vi "Periodic Tasks.vi"(8 "error in":errorcluster) -> ()   [LabVIEW 2017]
doc: "This VI runs in parallel to other robot code. It can contain as many user-defined periodic loops as you need. These can carry out PID or other sorts of timed response."
uses:
  <vilib>/Rock Robotics/WPI/Joystick/WPI_JoystickDeviceEnum.ctl
  <vilib>/Rock Robotics/WPI/Ultrasonic/WPI_SonarMB1010AnalogDeviceRef.ctl
  <vilib>/Rock Robotics/WPI/AnalogChannel/WPI_AnalogChannelDevRef.ctl
  <vilib>/Rock Robotics/SystemInterfaces/AI/FPGA_AIChannel.ctl
  <vilib>/Rock Robotics/WPI/ThirdParty/Sensors/ADIS16448 IMU/ADI_IMU_ADIS16448_IMUDevRef.ctl
  <vilib>/Rock Robotics/SystemInterfaces/spilib/spi_bus.ctl
  <vilib>/Rock Robotics/WPI/Utilities/WPI_GetSetVariantRefNum.vi
  <vilib>/Rock Robotics/WPI/Ultrasonic/WPI_SonarMB1010AnalogRefNum Registry Get.vi
  Robot Global Data.vi
  <vilib>/Rock Robotics/WPI/Ultrasonic/WPI_SonarMB1010AnalogGetRange.vi
  <vilib>/Rock Robotics/WPI/ThirdParty/Sensors/ADIS16448 IMU/ADIS16448_IMU.lvlib
panel:
  out "Current Faults":bool[](array[boolean])
  out "Battery Voltage Fault":bool
  out "Temperature Fault":bool
  out "Hardware Fault":bool
  out "IMU Angles Out":T1
  out "Z Angle":dbl
  out "Sonar Distance":dbl
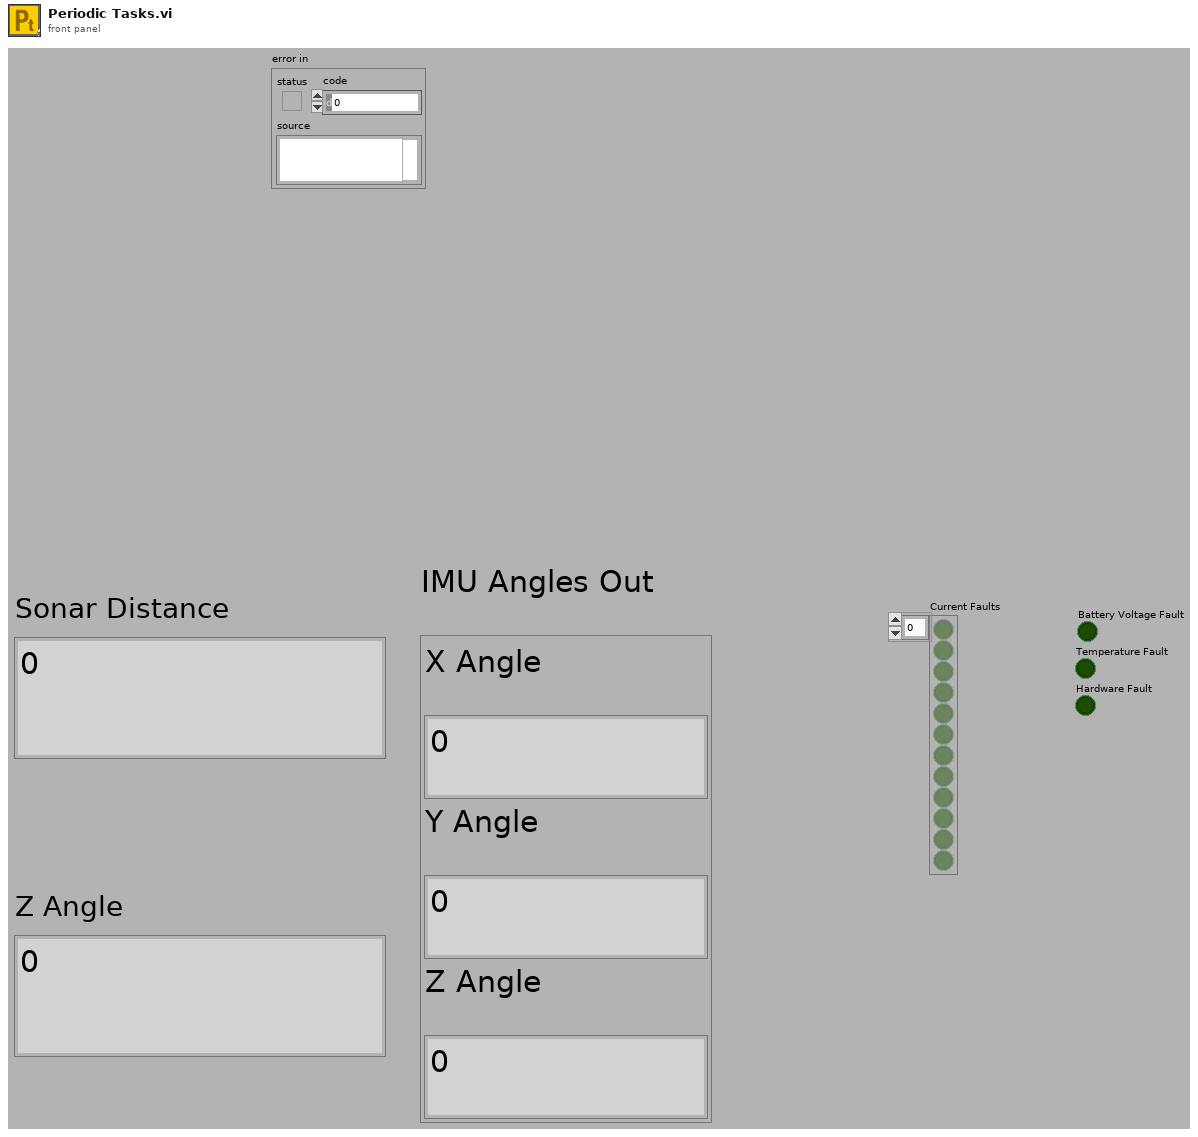
[diagram p1: front panel]
types:
  T1 = cluster{"X Angle":dbl, "Y Angle":dbl, "Z Angle":dbl}
  T2 = typedef "WPI_JoystickDeviceEnum.ctl" = enum16{"USB 0", "USB 1", "USB 2", "USB 3", "USB 4", "USB 5"}
  T3 = typedef "WPI_SonarMB1010AnalogDeviceRef.ctl" = cluster{"AIDeviceRef":T4, "Scaling factor (V/in)":dbl, "Average Bits":u8}
  T4 = typedef "WPI_AnalogChannelDevRef.ctl" = cluster{"DevStatus":errorcluster, "Analog Channel":T5}
  T5 = typedef "FPGA_AIChannel.ctl" = enum8{"AI 0", "AI 1", "AI 2", "AI 3", "AI MXP 0", "AI MXP 1", "AI MXP 2", "AI MXP 3", "Invalid"}
  T6 = typedef "ADIS16448_IMU.lvlib/ADI_IMU_ADIS16448_IMUDevRef.ctl" = cluster{"DevStatus":errorcluster, "Handle":i32, "SPI Bus":T7, "Device Found":bool, "Device Ready":bool, "Yaw Axis":enum16{"X", "Y", "Z"}, "AHRS Algorithm":enum16{"Complementary", "Madgwick"}, "Serial":u16, "Lot ID 2":u16, "Lot ID 1":u16, "Bytes Per Sample":u16, "Calibrate On Open?":bool}
  T7 = typedef "spi_bus.ctl" = enum16{"SPI On-Board, CS0", "SPI On-Board, CS1", "SPI On-Board, CS2", "SPI On-Board, CS3", "SPI MXP", "Invalid"}
  T8 = cluster{"Joystick 0":cluster{"Joystick 0":T2}, "Joystick 1":cluster{"Joystick 1":T2}, "Sonar":T3, "ADI IMU":T6}
  T9 = typedef "WPI_JoystickDevRef.ctl" = cluster{"Device":T2}
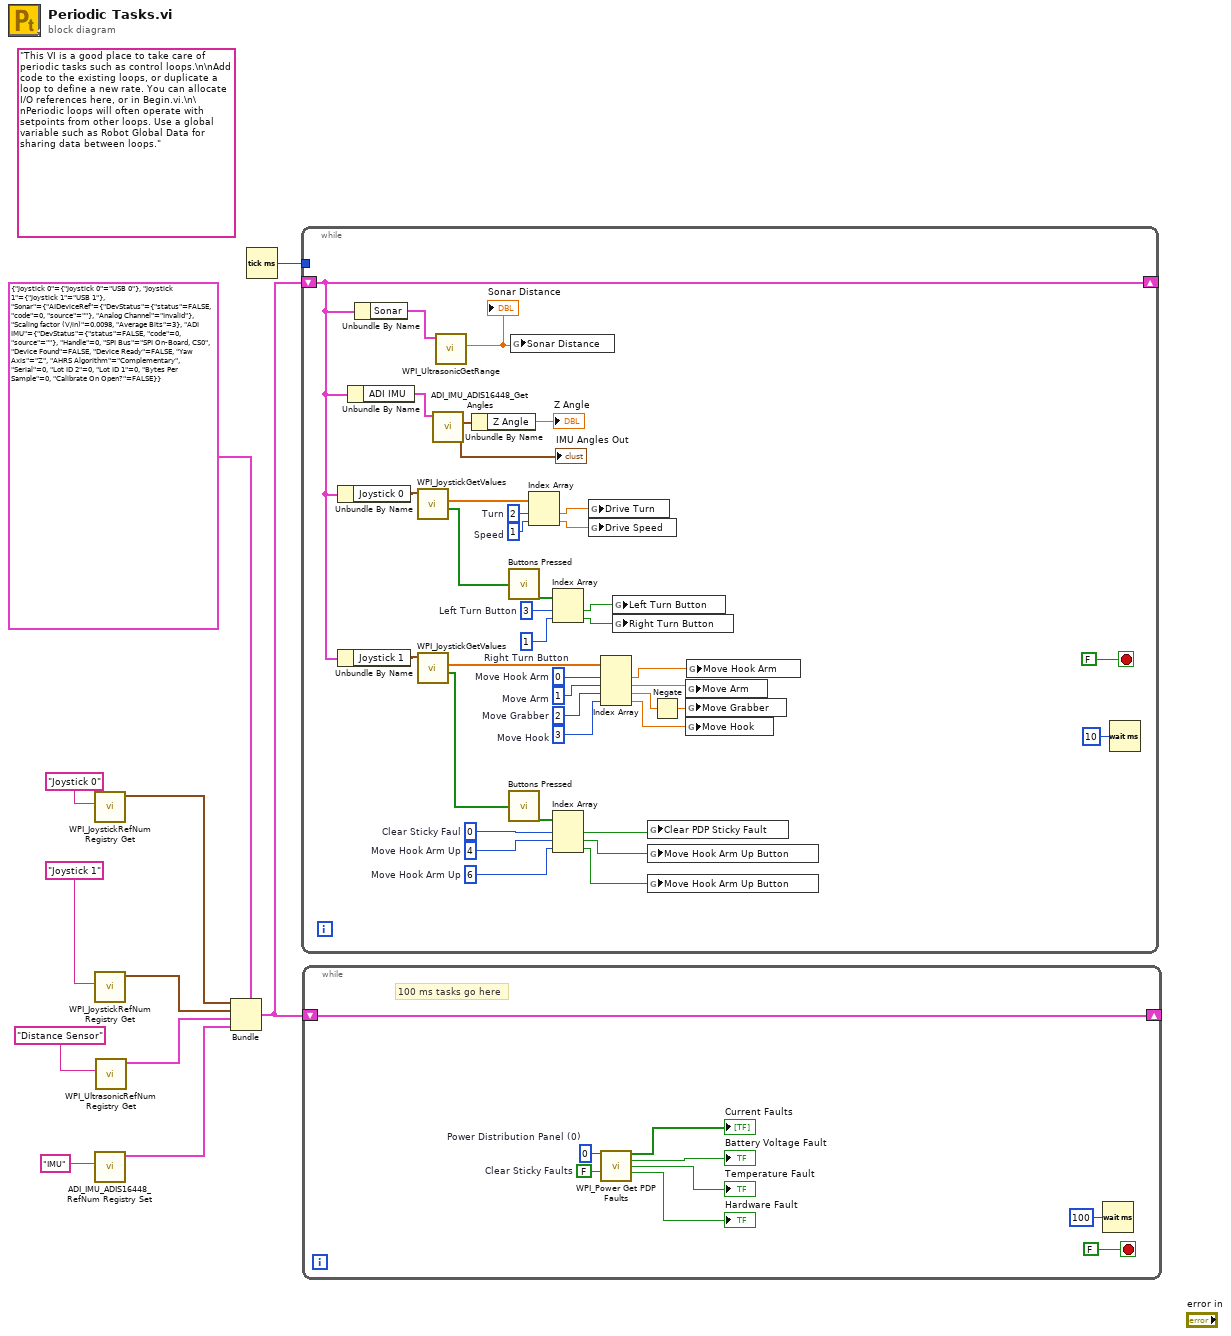
[diagram p0: block diagram]
diagram:
  (unwired) "This VI is a good place to take care of periodic tasks such as control loops.\n\nAdd code to the existing loops, or duplicate a loop to define a new rate. You can allocate I/O references here, or in Begin.vi.\n\nPeriodic loops will often operate with setpoints from other loops. Use a global variable such as Robot Global Data for sharing data between loops."
  n1 = call <vilib>:"WPI_JoystickRefNum Registry Get.vi"("refnum name"="Joystick 0") -> ("JoystickDevRef"=w8:T9)  [unwired: 1 in, 9 out]
  n2 = call <vilib>:"WPI_JoystickRefNum Registry Get.vi"("refnum name"="Joystick 1") -> ("JoystickDevRef"=w7:T9)  [unwired: 1 in, 9 out]
  n3 = call <vilib>:"ADI_IMU_ADIS16448_RefNum Registry Set.vi"("refnum name"="IMU") -> ("ADI IMU DevRef"=w1:T6)  [unwired: 9 in, 1 out]
  n4 = call-poly <vilib>:"WPI_UltrasonicRefNum Registry Get.vi"("refnum name"="Distance Sensor") -> ("SonarMB1010AnalogDevRef"=w2:T3)  [unwired: 9 in, 1 out]
  n5 = Bundle(cluster=T8 {"Joystick 0"={"Joystick 0"=enum."USB 0"}, "Joystick 1"={"Joystick 1"=enum."USB 1"}, "Sonar"={"AIDeviceRef"={"DevStatus"={"status"=FALSE, "code"=0, "source"=""}, "Analog Channel"=enum."Invalid"}, "Scaling factor (V/in)"=0.0098, "Average Bits"=3}, "ADI IMU"={"DevStatus"={"status"=FALSE, "code"=0, "source"=""}, "Handle"=0, "SPI Bus"=enum."SPI On-Board, CS0", "Device Found"=FALSE, "Device Ready"=FALSE, "Yaw Axis"=enum."Z", "AHRS Algorithm"=enum."Complementary", "Serial"=0, "Lot ID 2"=0, "Lot ID 1"=0, "Bytes Per Sample"=0, "Calibrate On Open?"=FALSE}}, "Joystick 0"=w8, "Joystick 1"=w7, "Sonar"=w2, "ADI IMU"=w1) -> (w6:T8)
  n6 = Tick Count (ms)() -> (millisecond timer value=w10:u32)
  n7 = while {
    shift-right: [w32] -> _
    shift-left: w6 -> [w32]
    tunnel: w10 -> [_]
    stop <- FALSE stop-if-true
    w13 = 6  # Move Hook Arm Up
    w15 = 4  # Move Hook Arm Up
    w26 = 3  # Move Hook
    w27 = 2  # Move Grabber
    w28 = 1  # Move Arm
    w29 = 0  # Move Hook Arm
    w30 = 1  # Speed
    w31 = 2  # Turn
    w36 = i8 0  # Clear Sticky Faul
    w41 = i8 1  # Right Turn Button
    w42 = i8 3  # Left Turn Button
    n8 = Unbundle By Name(w32) -> ("Joystick 0"=w38:cluster{"Joystick 0":T2})
    n9 = Unbundle By Name(w32) -> ("Joystick 1"=w37:cluster{"Joystick 1":T2})
    n10 = Unbundle By Name(w32) -> ("ADI IMU"=w39:T6)
    n11 = Unbundle By Name(w32) -> ("Sonar"=w40:T3)
    n12 = call <vilib>:"WPI_JoystickGetValues.vi"("JoystickDevRef"=w38) -> ("Buttons"=w44:bool[], "Axes"=w45:dbl[])  [unwired: 6 in, 3 out]
    n13 = call <vilib>:"WPI_JoystickGetValues.vi"("JoystickDevRef"=w37) -> ("Buttons"=w34:bool[], "Axes"=w33:dbl[])  [unwired: 6 in, 3 out]
    n14 = call <vilib>:"ADI_IMU_ADIS16448_Get Angles.vi"("ADI IMU DevRef"=w39) -> ("IMU Angles Out"=w47:T1)  [unwired: 7 in, 3 out]
    "IMU Angles Out" <- w47
    n15 = call-poly <vilib>:"WPI_UltrasonicGetRange.vi"("SonarMB1010AnalogDevRef"=w40) -> ("Distance"=w48:dbl)  [unwired: 8 in, 2 out]
    "Sonar Distance" <- w48
    n16 = Unbundle By Name(w47) -> ("Z Angle"=→"Z Angle":dbl)
    n17 = call "Buttons Pressed.vi"("Button Values"=w44) -> ("Button Presses"=w43:bool[])
    n18 = call "Buttons Pressed.vi"("Button Values"=w34) -> ("Button Presses"=w35:bool[])
    n19 = global write "Robot Global Data.vi" "Sonar Distance"(w48) -> ()
    n20 = Index Array(array=w45, index #1=w31, index #2=w30) -> (element #1=w22:dbl, element #2=w21:dbl)
    n21 = Index Array(array=w43, index #1=w42, index #2=w41) -> (element #1=w20:bool, element #2=w19:bool)
    n22 = Index Array(array=w35, index #1=w36, index #2=w15, index #3=w13) -> (element #1=w16:bool, element #2=w14:bool, element #3=w12:bool)
    n23 = global write "Robot Global Data.vi" "Drive Turn"(w22) -> ()
    n24 = global write "Robot Global Data.vi" "Drive Speed"(w21) -> ()
    n25 = Index Array(array=w33, index #1=w29, index #2=w28, index #3=w27, index #4=w26) -> (element #1=w17:dbl, element #2=w25:dbl, element #3=w24:dbl, element #4=w23:dbl)
    n26 = global write "Robot Global Data.vi" "Left Turn Button"(w20) -> ()
    n27 = global write "Robot Global Data.vi" "Right Turn Button"(w19) -> ()
    n28 = global write "Robot Global Data.vi" "Clear PDP Sticky Fault"(w16) -> ()
    n29 = global write "Robot Global Data.vi" "Move Hook Arm Up Button"(w14) -> ()
    n30 = global write "Robot Global Data.vi" "Move Hook Arm Up Button"(w12) -> ()
    n31 = Negate(x=w24) -> (-x=w18:dbl)
    n32 = global write "Robot Global Data.vi" "Move Arm"(w25) -> ()
    n33 = global write "Robot Global Data.vi" "Move Grabber"(w18) -> ()
    n34 = global write "Robot Global Data.vi" "Move Hook"(w23) -> ()
    n35 = global write "Robot Global Data.vi" "Move Hook Arm"(w17) -> ()
    n36 = Wait (ms)(milliseconds to wait=u32 10) -> ()  [unwired: 1 out]
  }
  n37 = while {
    shift-right: [w57] -> _
    shift-left: w6 -> [w57]
    stop <- FALSE stop-if-true
    w55 = FALSE  # Clear Sticky Faults
    w56 = u8 0  # Power Distribution Panel (0)
    # "100 ms tasks go here"
    n38 = call <vilib>:"WPI_Power Get PDP Faults.vi"("Power Distribution Panel (0)"=w56, "Clear Sticky Faults"=w55) -> ("Current Faults"=→"Current Faults":bool[], "Battery Voltage Fault"=→"Battery Voltage Fault":bool, "Temperature Fault"=→"Temperature Fault":bool, "Hardware Fault"=→"Hardware Fault":bool)  [unwired: 9 in, 1 out]
    n39 = Wait (ms)(milliseconds to wait=u32 100) -> ()  [unwired: 1 out]
  }
